vi "Init.vi"(8 "error in (no error)":errorcluster) -> (0 "error out":errorcluster, 3 "Test Group Manager out":refnum<class "Test Group Manager.lvclass">)   [LabVIEW 2016, in "Test Group Manager.lvlib" / "Test Group Manager.lvclass"]
uses:
  Test Group Manager.lvclass
  Test Group Manager.lvclass/Test Group Manager.ctl
  Protected Methods/Write Test Group Database.vi
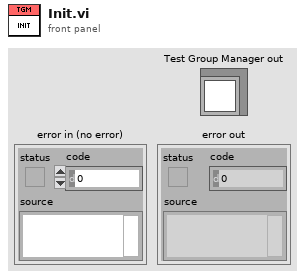
[diagram p1: front panel]
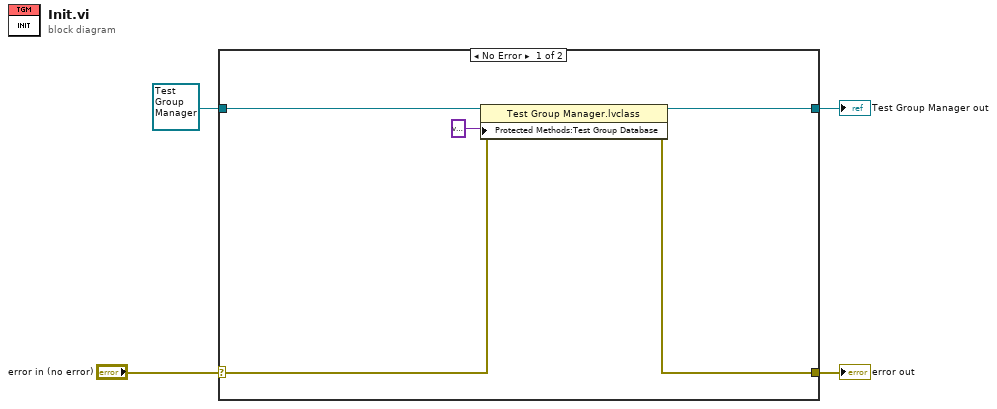
[diagram p0: block diagram]
diagram:
  n1 = case shown="No Error" "error in (no error)" {
    selector: "error in (no error)" -> [w9 w11]
    tunnel: [w8 w11] -> w3
    tunnel: [w6 w10] -> w1
    tunnel: refnum<class "Test Group Manager.lvclass"> refnum ("Test Group Manager in") -> [w7 w10]
    frame No Error {
      n2 = property class="Test Group Manager.lvclass"(reference=w7, error in=w9, "Protected Methods:Test Group Database"=variant ("Test Group Database")) -> (reference out=w6:refnum<class "Test Group Manager.lvclass">, error out=w8:errorcluster)
    }
    frame Error {
    }
  }
  "error out" <- w3
  "Test Group Manager out" <- w1
